vi "Pre_Loop.vi"(8 "Error In":errorcluster, 11 "This VI":refnum<vi>) -> (0 "Error Out":errorcluster, 3 "Event Registration Refnum":refnum<event-registration>)   [LabVIEW 2020]
doc: "This is where need to be all the things that must be set before the loops. The start of the module (queue that sends the start) is also inside."
uses:
  User Events/Controls/UEA_Action.ctl
  Queue/Controls/Queue.ctl
  Queue/Controls/Queue_Mode.ctl
  Queue/Controls/Queue_Action.ctl
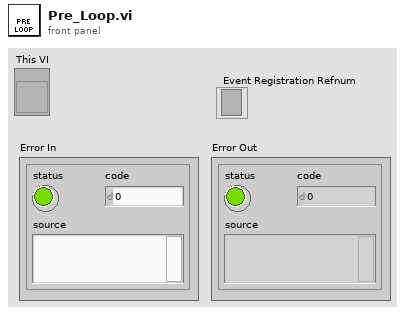
[diagram p1: front panel]
types:
  T1 = typedef "Queue_Action.ctl" = enum16{"Get", "Set", "Release"}
  T2 = typedef "Queue.ctl" = cluster{"Mode":T3, "Data":variant}
  T3 = typedef "Queue_Mode.ctl" = enum16{"Start", "Stop"}
  T4 = typedef "UEA_Action.ctl" = enum16{"Create", "Get", "Destroy"}
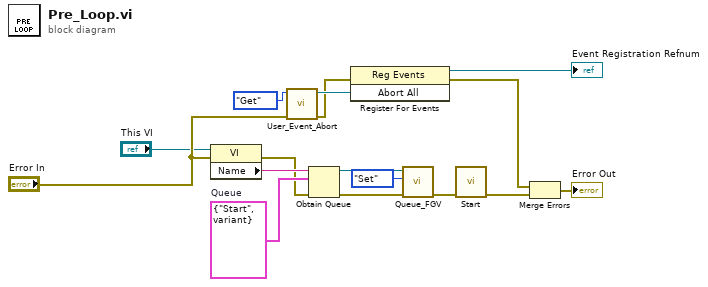
[diagram p0: block diagram]
diagram:
  w10 = T2 {"Mode"=enum."Start", "Data"=variant}  # Queue
  n1 = property class="VI"(reference="This VI", error in="Error In") -> (error out=w7:errorcluster, "Name"=w11:string)  [unwired: 1 out]
  n2 = call "User_Event_Abort.vi"("Error In"="Error In", "Action"=UEA_Action."Get") -> ("Error Out"=w14:errorcluster, "Abort All"=w16:refnum<user-event>)  [unwired: 8 in]
  n3 = Obtain Queue(name (unnamed)=w11, element data type=w10, error in (no error)=w7) -> (queue out=w9:refnum<queue>, error out=w8:errorcluster)  [unwired: 2 in, 1 out]
  n4 = register-events(error in=w14, w16) -> (reference out=→"Event Registration Refnum":refnum<event-registration>, error out=w12:errorcluster)  [unwired: 1 in]
  n5 = call "Queue_FGV.vi"("error in"=w8, "Action"=Queue_Action."Set", "Queue In"=w9) -> ("error out"=w3:errorcluster)  [unwired: 7 in, 1 out]
  n6 = call "Start.vi"("error in"=w3) -> ("error out"=w2:errorcluster)  [unwired: 10 in]
  n7 = Merge Errors(w12, w2) -> (→"Error Out":errorcluster)
